vi "Actor Core.vi"(8 "error in":errorcluster, 11 "Diagnostic in":refnum<class "Diagnostic.lvclass">) -> (0 "error out":errorcluster={"status"=TRUE, "code"=1556, "source"="In Place Element Structure in Actor Framework.lvlib:Message Priority Queue.lvclass:Priority Dequeue.vi:2780001->Actor Framework.lvlib:Actor.lvclass:Actor Core.vi:5880002->Diagnostic.lvlib:Diagnostic.lvclass:Actor Core.vi"}, 3 "Actor out":refnum<class "Actor.lvclass">)   [LabVIEW 2023, in "GUI.lvlib" / "Diagnostic.lvlib" / "Diagnostic.lvclass"]
doc: "(<B>Filename</B>: Actor Framework.lvlib:Actor.lvclass:Actor Core.vi)\n\nReceives messages to the actor, reacts to them, and initiates any error handling that may shut the actor down.\n\nDescendant classes may override this VI to append parallel tasks for the actor to complete while it handles messages. Overrides use the Call Parent Method node."
uses:
  Diagnostic.lvclass
  <vilib>/ActorFramework/Actor/Actor.lvclass
  C:/Program Files/National Instruments/LabVIEW 2023/vi.lib/ActorFramework/Actor/Actor.lvclass
  <vilib>/ActorFramework/Actor/Actor.lvclass/Actor.ctl
  <vilib>/ActorFramework/Message Enqueuer/Message Enqueuer.lvclass/Message Enqueuer.ctl
  Reused Code/Subpanels Actor/subpanels/subpanel Messages/Insert Msg/Insert Msg.lvclass/Insert Msg.ctl
  Diagnostic Messages/Call Instruments Msg/Call Instruments Msg.lvclass/Call Instruments Msg.ctl
  Diagnostic Messages/Global Reset Msg/Global Reset Msg.lvclass/Global Reset Msg.ctl
  <vilib>/ActorFramework/Message Enqueuer/Init from Existing Queue.vi
  <vilib>/ActorFramework/Message Enqueuer/Enqueue.vi
  Reused Code/Subpanels Actor/subpanels/subpanel Messages/Insert Msg/Insert Msg.lvclass
  C:/Program Files/National Instruments/LabVIEW 2023/vi.lib/ActorFramework/Message/Message.lvclass
  Diagnostic Messages/Call Instruments Msg/Call Instruments Msg.lvclass
  Diagnostic Messages/Global Reset Msg/Global Reset Msg.lvclass
  <vilib>/ActorFramework/Message Priority Queue/Priority Enqueue.vi
  <vilib>/ActorFramework/Message Enqueuer/Message Enqueuer.lvclass
  Reused Code/Subpanels Actor/subpanels/subpanel/subpanel (abstract).lvclass
  Diagnostic.lvclass/Diagnostic.ctl
  HardwareAbstractionLayer_LVOOP/Error Handler/Error Handler_class/Error Handler.lvclass
panel:
  in  "Call NI DMM":bool
  in  "Call Scope":bool
  in  "Call FGEN":bool
  in  "Call Relay Output":bool
  in  "Call Waveform Generation":bool
  in  "Call PPS":bool
  in  "Call Analog Output":bool
  in  "Call Analog Input":bool
  in  "Call Digital Output":bool
  in  "Call Digital Input":bool
  in  "Call Database":bool
  in  "Call Scanner":bool
  in  "Call RS485":bool
  in  "Call NI PWM Input":bool
  in  "Call CAN":bool
  in  "Call NI PWM Output":bool
  in  "Global Reset":bool
  in  "Stop":bool=TRUE
  # "Digital"
  # "CAN"
  # "Power Supply"
  # "Analog"
  # "PWM"
  # "Temparature Controller"
  # "Scanner"
  # "NI Instruments"
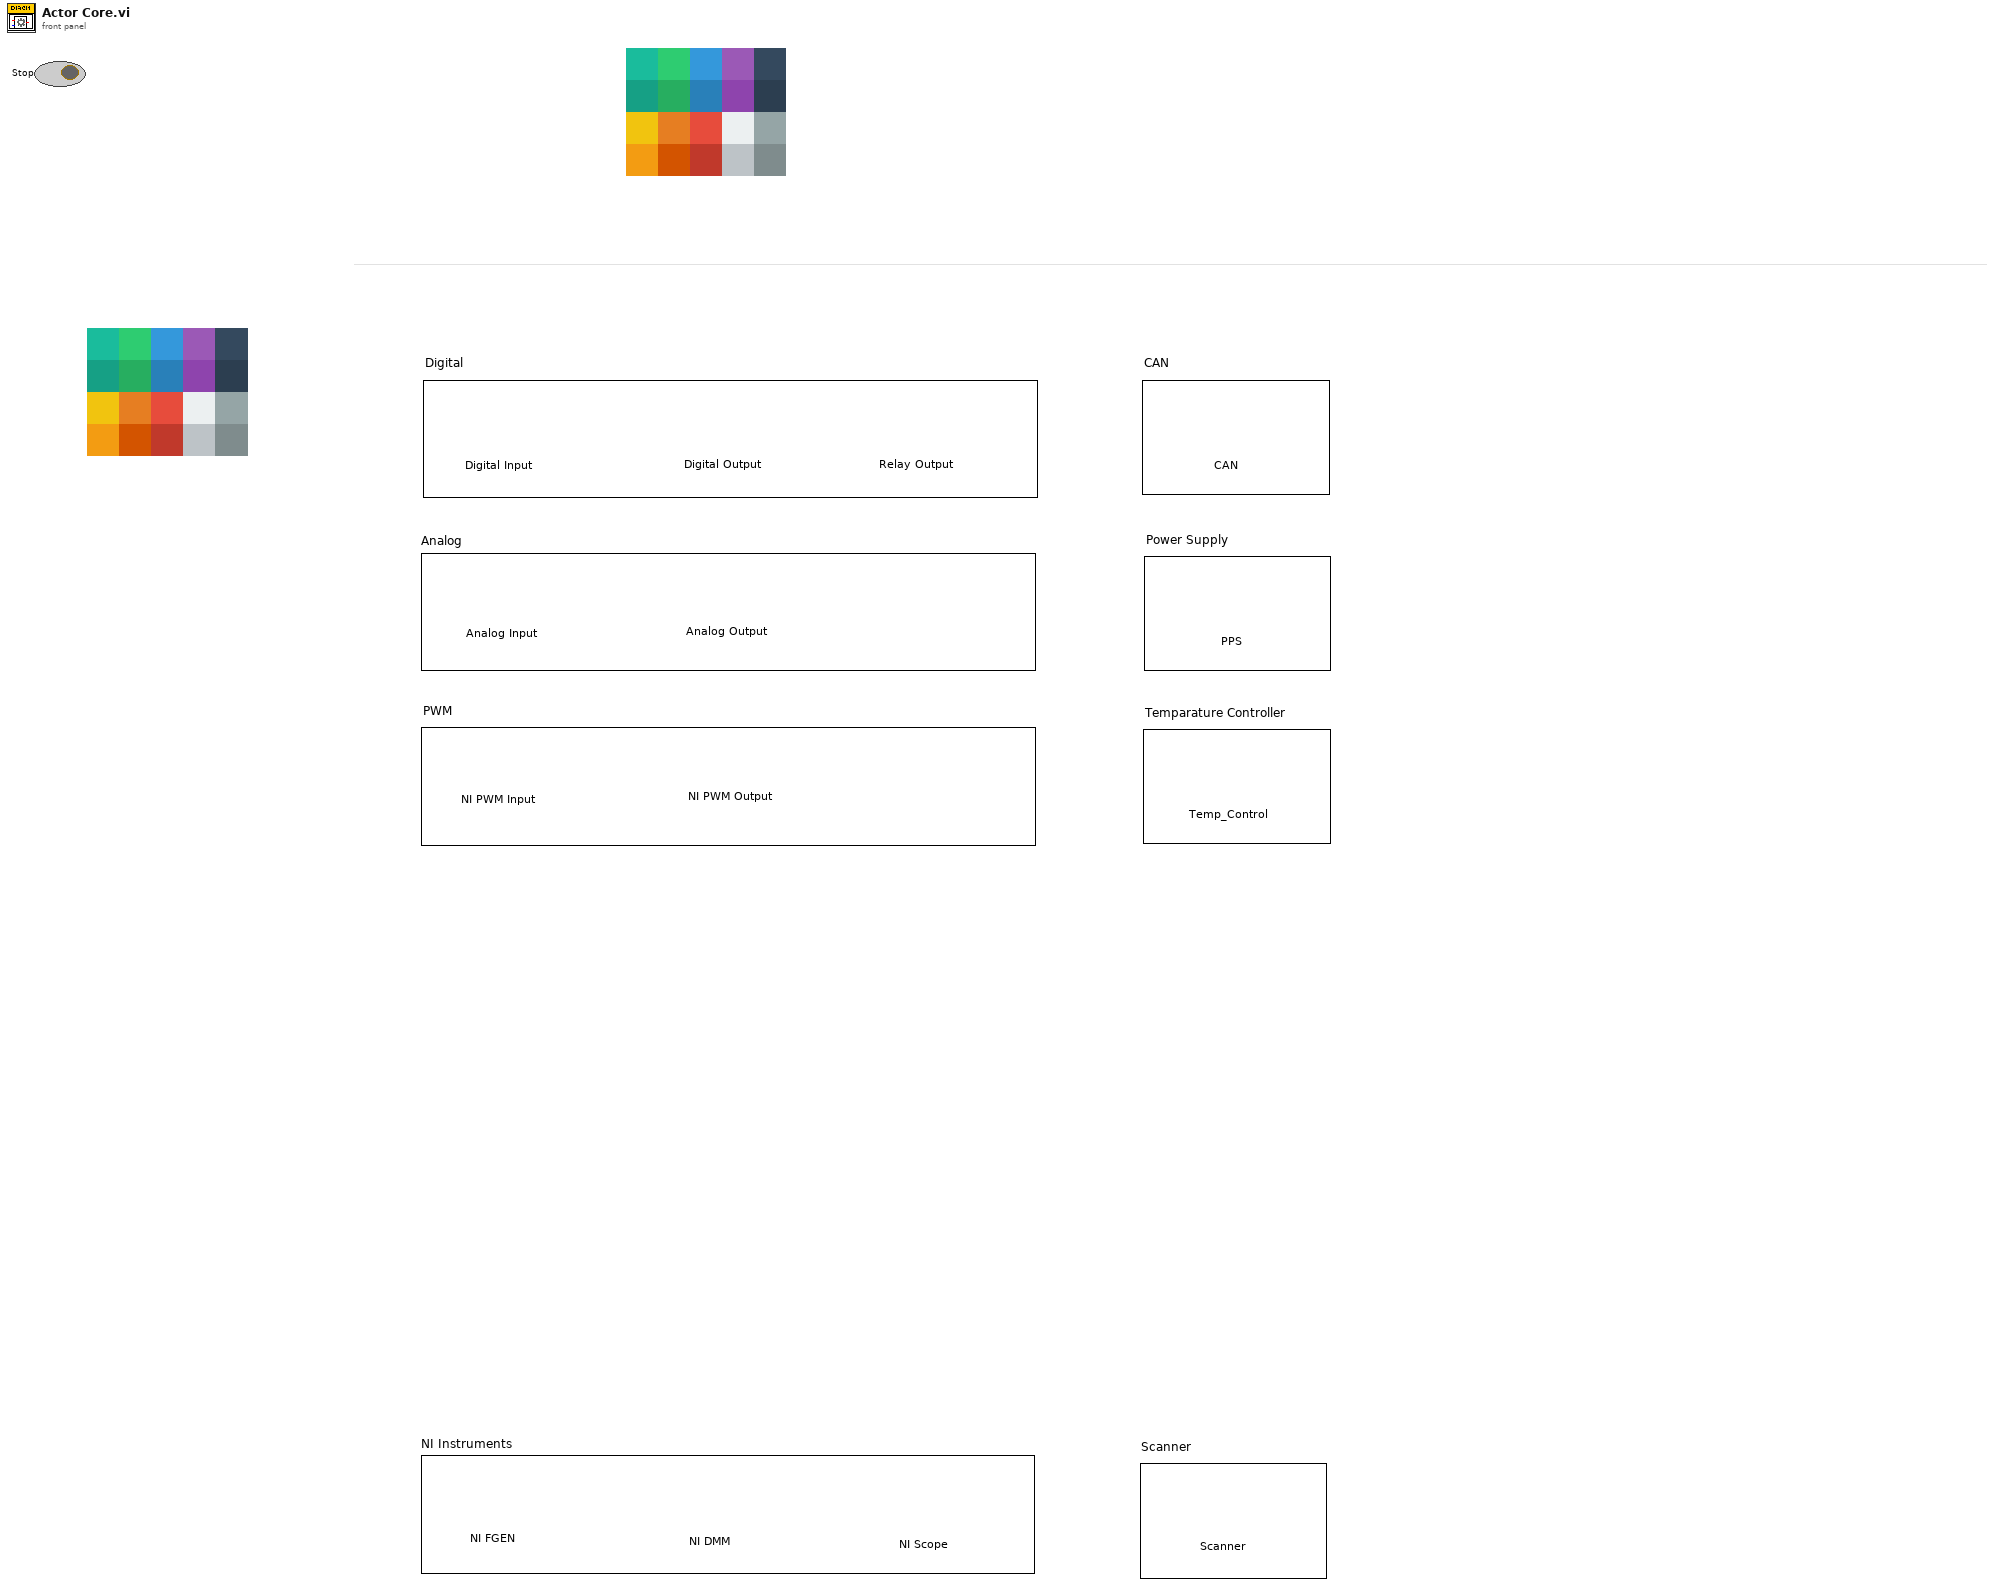
[diagram p1: front panel]
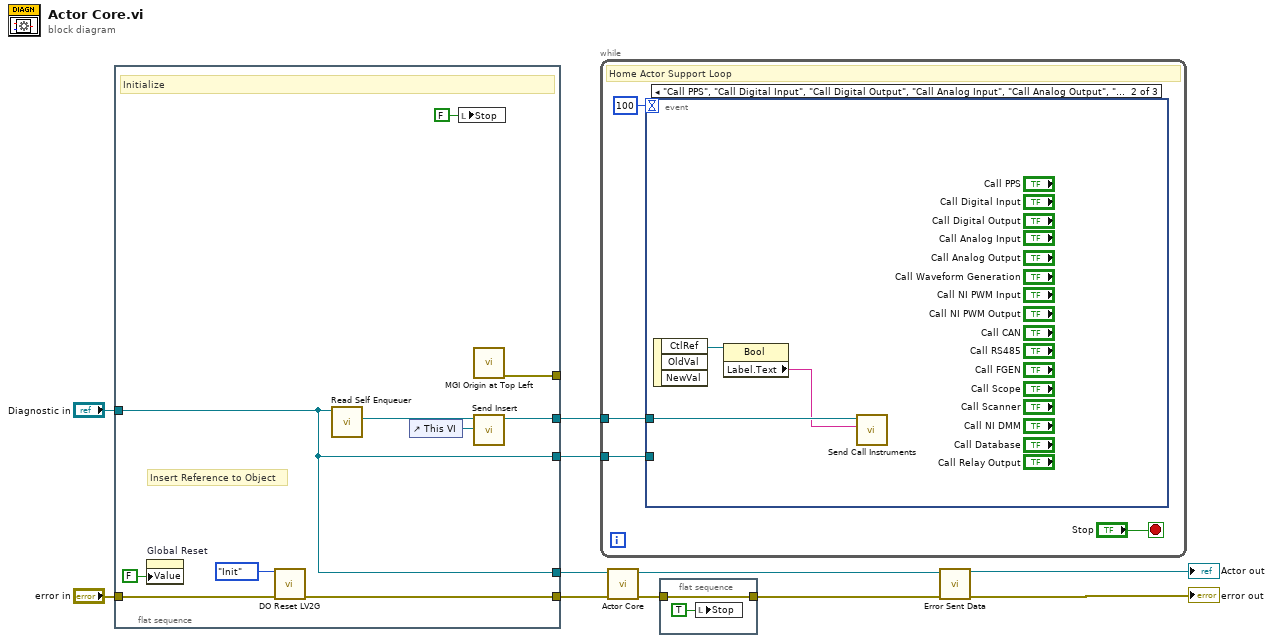
[diagram p0: block diagram]
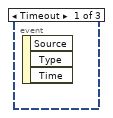
[diagram p2: hidden frame]
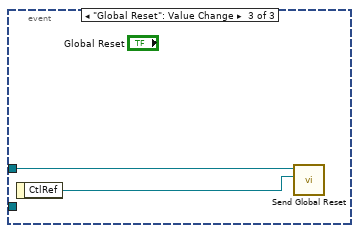
[diagram p3: hidden frame]
diagram:
  n1 = flat-sequence {
    tunnel: "Diagnostic in" -> [w19]
    tunnel: [w17] -> w3
    tunnel: [w19] -> w9
    tunnel: [w12] -> w8
    tunnel: "error in" -> [w13]
    tunnel: [w20] -> _
    tunnel: [w19] -> w7
    frame #0 {
      # "Insert Reference to Object"
      # "Initialize"
      n2 = property on="Global Reset" class="Bool (strict)"("Value"=FALSE ("Global Reset")) -> ()  [unwired: 2 in, 2 out]
      n3 = call "DO Reset LV2G.vi"("Task"=enum16{"Init", "Write", "Read"}."Init", "error in"=w13) -> ("error out"=w12:errorcluster)  [unwired: 10 in, 3 out]
      n4 = call <vilib>:"Read Self Enqueuer.vi"("Actor"=w19) -> ("Self Enqueuer"=w18:refnum<class "Message Enqueuer.lvclass">)  [unwired: 10 in]
      n5 = control-ref of="This VI"() -> (w16:refnum<vi>)
      n6 = local write "Stop"(FALSE ("Stop")) -> ()
      n7 = call <userlib>:"MGI Origin at Top Left.vi"() -> ("Error Out"=w20:errorcluster)  [unwired: 9 in, 1 out]
      n8 = call "Send Insert.vi"("VI Ref"=w16, "Message Enqueuer"=w18) -> ("Message Enqueuer out"=w17:refnum<class "Message Enqueuer.lvclass">)  [unwired: 8 in, 1 out]
    }
  }
  n9 = while {
    tunnel: w3 -> [w22]
    tunnel: w7 -> [w21]
    stop <- "Stop" stop-if-true
    # "Home Actor Support Loop"
    n10 = event shown="[1] \"Call PPS\", \"Call Digital Input\", \"Call Digital Output\", \"Call Analog Input\", \"Call Analog Output\", \"Call Waveform Generation\", \"Call NI PWM Input\", \"Call NI PWM Output\", \"Call CAN\", \"Call RS485\", \"Call Scanner\", \"Call NI DMM\", \"Call Scope\", \"Call FGEN\", \"Call Database\", \"Call Relay Output\": Value Change" {
      selector: _ -> [_ _ _]
      dyn-events: _ -> [_ _ _]
      timeout: 100 -> [_ _ _]
      tunnel: w22 -> [_ w27 w29]
      tunnel: w21 -> [_ _ _]
      event Timeout {
        n11 = event-data() -> ()  [unwired: 1 in, 3 out]
      }
      event "Call PPS", "Call Digital Input", "Call Digital Output", "Call Analog Input", "Call Analog Output", "Call Waveform Generation", "Call NI PWM Input", "Call NI PWM Output", "Call CAN", "Call RS485", "Call Scanner", "Call NI DMM", "Call Scope", "Call FGEN", "Call Database", "Call Relay Output": Value Change {
        n12 = event-data() -> ("CtlRef"=w26:refnum<vi>)  [unwired: 1 in, 2 out]
        n13 = property class="Bool"(reference=w26) -> ("Label.Text"=w25:string)  [unwired: 1 in, 2 out]
        n14 = call "Send Call Instruments.vi"("Instrument?"=w25, "Message Enqueuer"=w27) -> ()  [unwired: 8 in, 2 out]
      }
      event "Global Reset": Value Change {
        n15 = event-data() -> ("CtlRef"=w28:refnum<vi>)  [unwired: 1 in]
        n16 = call "Send Global Reset.vi"("Clobal Reset"=w28, "Message Enqueuer"=w29) -> ()  [unwired: 8 in, 2 out]
      }
    }
  }
  n17 = call-parent "Actor Core.vi"("error in"=w8, "Actor in"=w9) -> ("error out"=w10:errorcluster, "Actor out"=→"Actor out":refnum<class "Actor.lvclass">)  [unwired: 8 in]
  n18 = flat-sequence {
    tunnel: w10 -> [w31]
    tunnel: [w31] -> w2
    frame #0 {
      n19 = local write "Stop"(TRUE ("Stop")) -> ()
    }
  }
  n20 = call "Error Sent Data.vi"("error in"=w2) -> ("error out"=→"error out":errorcluster)  [unwired: 10 in]
